vi "回正判定.vi"(0 "曲线引用":refnum<vi>, 1 "回正判定":T1, 3 "错误输入":errorcluster) -> (7 "曲线引用输出":refnum<vi>, 8 "OK":bool, 10 "错误输出":errorcluster)   [LabVIEW 2018]
uses:
  Global_Variable/Global.vi
  Global_Variable/A180648.vi
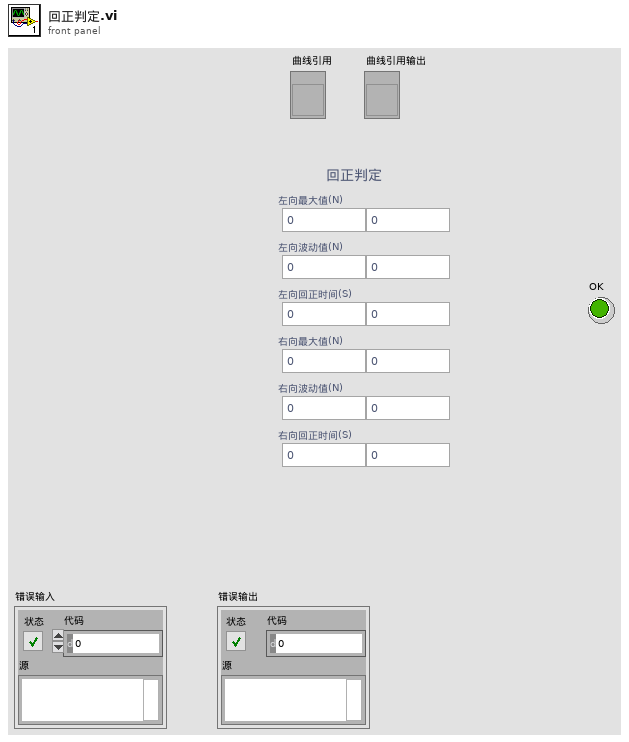
[diagram p1: front panel]
types:
  T1 = cluster{"左向最大值(N)":cluster{"下限":dbl, "上限":dbl}, "左向波动值(N)":cluster{"下限":dbl, "上限":dbl}, "左向回正时间(S)":cluster{"下限":dbl, "上限":dbl}, "右向最大值(N)":cluster{"下限":dbl, "上限":dbl}, "右向波动值(N)":cluster{"下限":dbl, "上限":dbl}, "右向回正时间(S)":cluster{"下限":dbl, "上限":dbl}}
  T2 = enum32{"空载", "功能", "力特性", "传感器特性", "电流特性", "振动NVH", "逆向空载", "完成"}
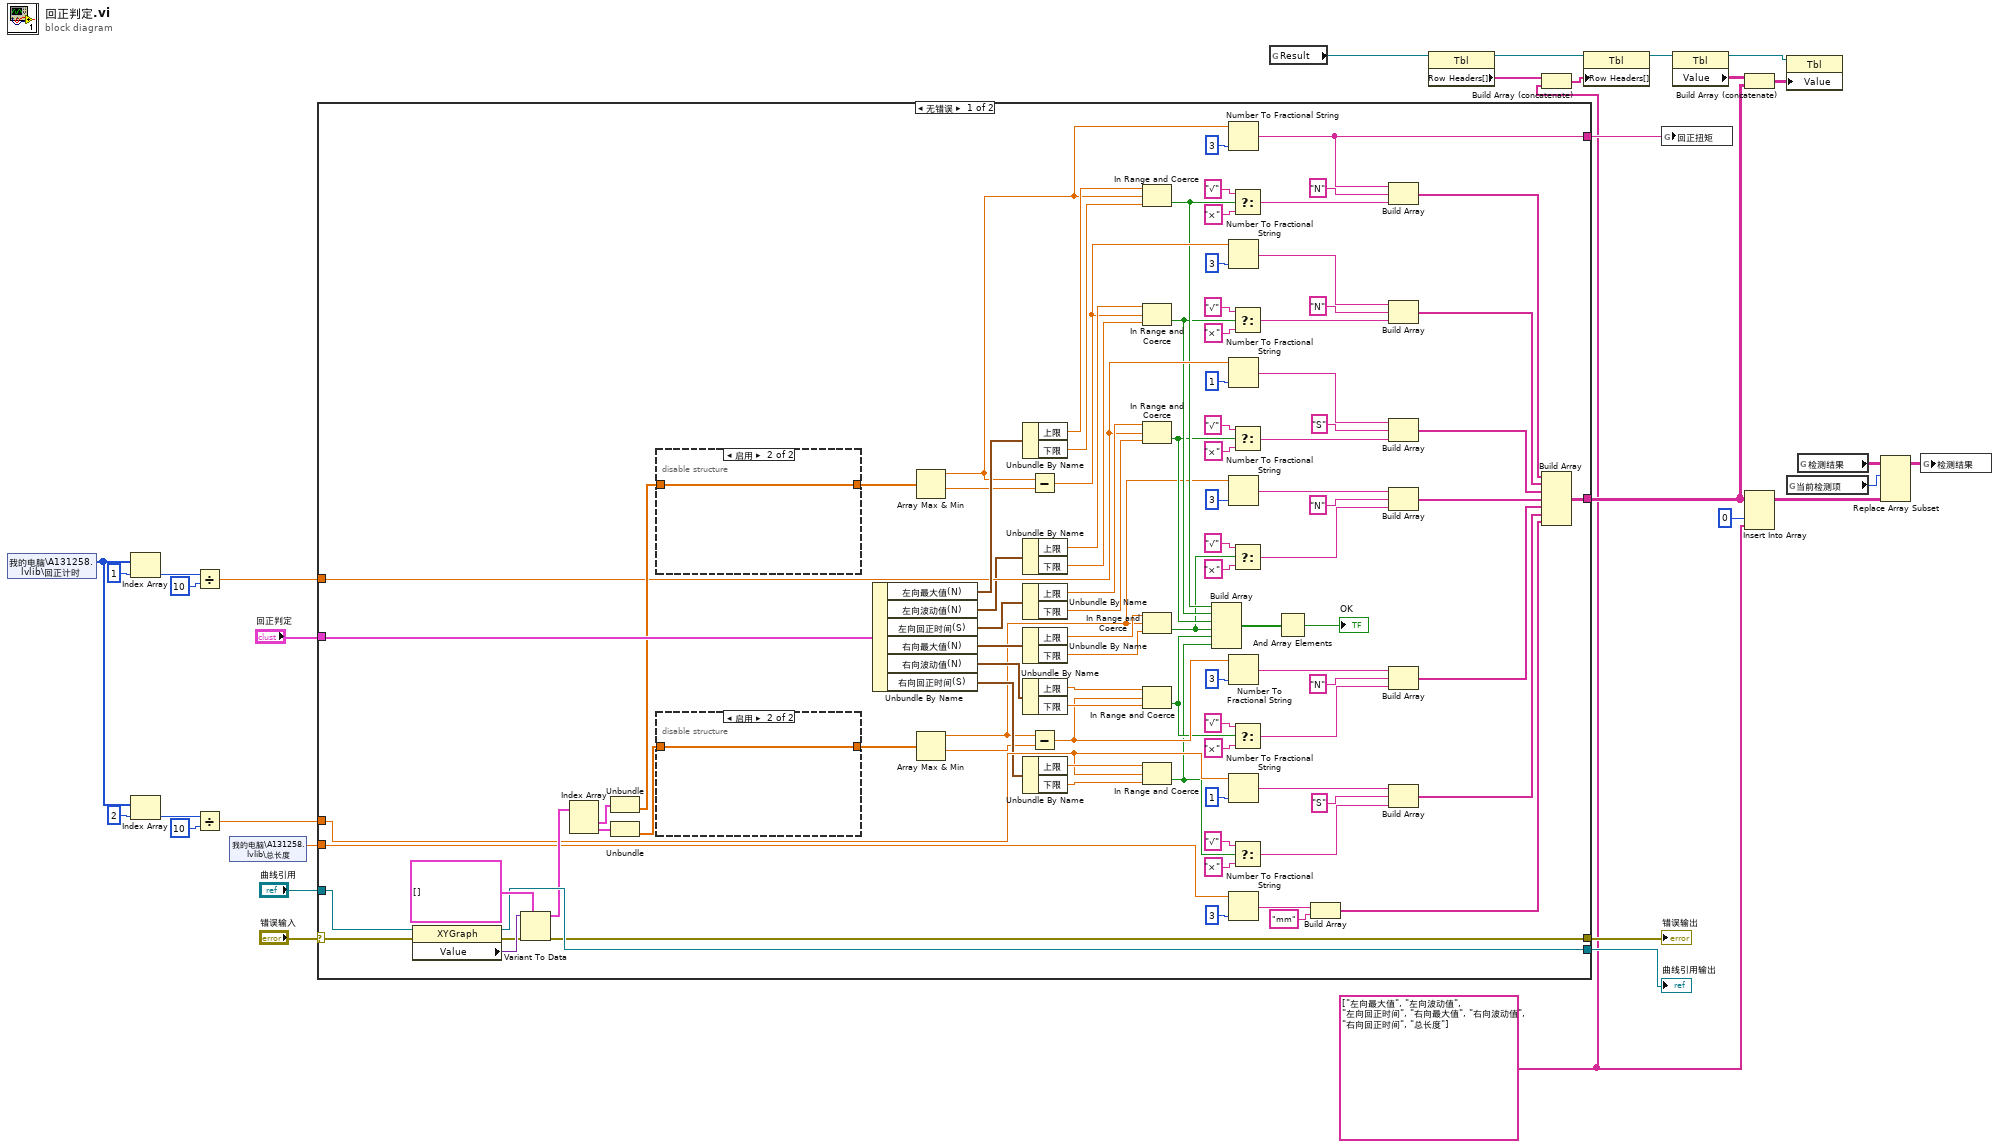
[diagram p0: block diagram]
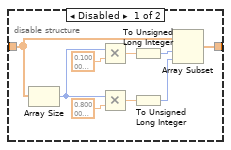
[diagram p2: hidden frame]
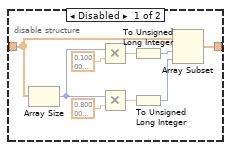
[diagram p3: hidden frame]
diagram:
  w3 = string[] ["左向最大值", "左向波动值", "左向回正时间", "右向最大值", "右向波动值", "右向回正时间", "总长度"] ("元素")
  n1 = shared-variable "我的电脑\\A131258.lvlib\\回正计时"() -> (w15:u32[])  [unwired: 1 in, 1 out]
  n2 = Index Array(array=w15, index=1 ("索引")) -> (element=w13:u32)
  n3 = Index Array(array=w15, index=2 ("索引")) -> (element=w10:u32)
  n4 = Divide(x=w13, y=u32 10) -> (x/y=w14:dbl)
  n5 = Divide(x=w10, y=u32 10) -> (x/y=w9:dbl)
  n6 = shared-variable "我的电脑\\A131258.lvlib\\总长度"() -> (w8:sgl)  [unwired: 1 in, 1 out]
  n7 = case shown="无错误" "错误输入" {
    selector: "错误输入" -> [w126 w150]
    tunnel: [w122 w150] -> w30
    tunnel: "曲线引用" -> [w125 w149]
    tunnel: [w124 w149] -> w28
    tunnel: "回正判定" -> [w118 _]
    tunnel: [w101 _] -> w4
    tunnel: [w96 _] -> w19
    tunnel: w14 -> [w55 _]
    tunnel: w9 -> [w54 _]
    tunnel: w8 -> [w34 _]
    frame No Error {
      n8 = property class="XYGraph"(reference=w125, error in=w126) -> (reference out=w124:refnum<vi>, error out=w123:errorcluster, "Value"=w128:variant)
      n9 = Variant To Data(error in=w123, type=cluster{dbl[], dbl[]}[] [], Variant=w128) -> (data=w121:cluster{dbl[], dbl[]}[], error out=w122:errorcluster)
      n10 = Index Array(array=w121) -> (element #1=w120:cluster{dbl[], dbl[]}, element #2=w119:cluster{dbl[], dbl[]})  [unwired: 2 in]
      n11 = Unbundle(w120) -> (w63:dbl[])  [unwired: 1 out]
      n12 = Unbundle(w119) -> (w62:dbl[])  [unwired: 1 out]
      n13 = disable-structure shown="启用" {
        disable-tunnel: [w147 w148] -> w99
        disable-tunnel: w63 -> [w139 w148]
        frame Disabled {
          n14 = Array Size(array=w139) -> (size(s)=w140:i32)
          n15 = Multiply(x=w140, y=sgl 0.1) -> (x*y=w144:sgl)
          n16 = Multiply(x=w140, y=sgl 0.8) -> (x*y=w145:sgl)
          n17 = To Unsigned Long Integer(number=w144) -> (unsigned 32bit integer=w146:u32)
          n18 = To Unsigned Long Integer(number=w145) -> (unsigned 32bit integer=w141:u32)
          n19 = Array Subset(array=w139, index=w146, length=w141) -> (w147:dbl[])
        }
        frame Enabled {
        }
      }
      n20 = disable-structure shown="启用" {
        disable-tunnel: [w137 w138] -> w100
        disable-tunnel: w62 -> [w129 w138]
        frame Disabled {
          n21 = Array Size(array=w129) -> (size(s)=w136:i32)
          n22 = Multiply(x=w136, y=sgl 0.1) -> (x*y=w132:sgl)
          n23 = Multiply(x=w136, y=sgl 0.8) -> (x*y=w131:sgl)
          n24 = To Unsigned Long Integer(number=w132) -> (unsigned 32bit integer=w130:u32)
          n25 = To Unsigned Long Integer(number=w131) -> (unsigned 32bit integer=w135:u32)
          n26 = Array Subset(array=w129, index=w130, length=w135) -> (w137:dbl[])
        }
        frame Enabled {
        }
      }
      n27 = Unbundle By Name(w118) -> ("左向最大值(N)"=w117:cluster{"下限":dbl, "上限":dbl}, "左向波动值(N)"=w53:cluster{"下限":dbl, "上限":dbl}, "左向回正时间(S)"=w52:cluster{"下限":dbl, "上限":dbl}, "右向最大值(N)"=w61:cluster{"下限":dbl, "上限":dbl}, "右向波动值(N)"=w51:cluster{"下限":dbl, "上限":dbl}, "右向回正时间(S)"=w50:cluster{"下限":dbl, "上限":dbl})
      n28 = Array Max & Min(array=w99) -> (max value=w60:dbl, min value=w59:dbl)  [unwired: 2 out]
      n29 = Array Max & Min(array=w100) -> (max value=w32:dbl, min value=w49:dbl)  [unwired: 2 out]
      n30 = Unbundle By Name(w117) -> ("上限"=w103:dbl, "下限"=w102:dbl)
      n31 = Unbundle By Name(w53) -> ("上限"=w93:dbl, "下限"=w94:dbl)
      n32 = Unbundle By Name(w52) -> ("上限"=w82:dbl, "下限"=w81:dbl)
      n33 = Unbundle By Name(w61) -> ("上限"=w98:dbl, "下限"=w97:dbl)
      n34 = Unbundle By Name(w51) -> ("上限"=w78:dbl, "下限"=w79:dbl)
      n35 = Unbundle By Name(w50) -> ("上限"=w65:dbl, "下限"=w64:dbl)
      n36 = Subtract(x=w60, y=w59) -> (x-y=w58:dbl)
      n37 = Subtract(x=w32, y=w49) -> (x-y=w48:dbl)
      n38 = In Range and Coerce(upper limit=w103, x=w60, lower limit=w102) -> (In Range?=w43:bool)  [unwired: 1 out]
      n39 = In Range and Coerce(upper limit=w93, x=w58, lower limit=w94) -> (In Range?=w42:bool)  [unwired: 1 out]
      n40 = In Range and Coerce(upper limit=w82, x=w55, lower limit=w81) -> (In Range?=w41:bool)  [unwired: 1 out]
      n41 = In Range and Coerce(upper limit=w98, x=w32, lower limit=w97) -> (In Range?=w40:bool)  [unwired: 1 out]
      n42 = In Range and Coerce(upper limit=w78, x=w48, lower limit=w79) -> (In Range?=w39:bool)  [unwired: 1 out]
      n43 = In Range and Coerce(upper limit=w65, x=w54, lower limit=w64) -> (In Range?=w38:bool)  [unwired: 1 out]
      n44 = Build Array(w43, w42, w41, w40, w39, w38) -> (w105:bool[])
      n45 = Number To Fractional String(number=w60, precision (6)=i16 3 ("精度(6)")) -> (F-format string=w96:string)  [unwired: 2 in]
      n46 = Number To Fractional String(number=w58, precision (6)=i16 3 ("精度(6)")) -> (F-format string=w95:string)  [unwired: 2 in]
      n47 = Number To Fractional String(number=w55, precision (6)=i16 1 ("精度(6)")) -> (F-format string=w80:string)  [unwired: 2 in]
      n48 = Number To Fractional String(number=w32, precision (6)=i16 3 ("精度(6)")) -> (F-format string=w107:string)  [unwired: 2 in]
      n49 = Number To Fractional String(number=w48, precision (6)=i16 3 ("精度(6)")) -> (F-format string=w76:string)  [unwired: 2 in]
      n50 = Number To Fractional String(number=w54, precision (6)=i16 1 ("精度(6)")) -> (F-format string=w67:string)  [unwired: 2 in]
      n51 = Number To Fractional String(number=w34, precision (6)=i16 3 ("精度(6)")) -> (F-format string=w36:string)  [unwired: 2 in]
      n52 = Select(t="√", s=w43, f="×") -> (s? t:f=w112:string)
      n53 = Select(t="√", s=w42, f="×") -> (s? t:f=w92:string)
      n54 = Select(t="√", s=w41, f="×") -> (s? t:f=w83:string)
      n55 = Select(t="√", s=w40, f="×") -> (s? t:f=w111:string)
      n56 = Select(t="√", s=w39, f="×") -> (s? t:f=w72:string)
      n57 = Select(t="√", s=w38, f="×") -> (s? t:f=w71:string)
      n58 = And Array Elements(Boolean array=w105) -> (logical AND=→"OK":bool)
      n59 = Build Array(w36, "mm" ("元素")) -> (w33:string[])
      n60 = Build Array(w96, "N" ("元素"), w112) -> (w57:string[])
      n61 = Build Array(w95, "N" ("元素"), w92) -> (w56:string[])
      n62 = Build Array(w80, "S" ("元素"), w83) -> (w47:string[])
      n63 = Build Array(w107, "N" ("元素"), w111) -> (w46:string[])
      n64 = Build Array(w76, "N" ("元素"), w72) -> (w45:string[])
      n65 = Build Array(w67, "S" ("元素"), w71) -> (w44:string[])
      n66 = Build Array(w57, w56, w47, w46, w45, w44, w33) -> (w101:string[][])
    }
    frame Error {
    }
  }
  "错误输出" <- w30
  "曲线引用输出" <- w28
  n67 = global read "Global.vi" "Result"() -> (w27:refnum<vi>)
  n68 = property class="Tbl"(reference=w27) -> (reference out=w24:refnum<vi>, "Row Headers[]"=w26:string[])  [unwired: 1 in, 1 out]
  n69 = Build Array (concatenate)(w26, w3) -> (w25:string[])
  n70 = property class="Tbl"(reference=w24, "Row Headers[]"=w25) -> (reference out=w23:refnum<vi>)  [unwired: 1 in, 1 out]
  n71 = global write "检测结果.vi" "回正扭矩"(w19) -> ()
  n72 = property class="Tbl"(reference=w23) -> (reference out=w22:refnum<vi>, "Value"=w21:string[][])  [unwired: 1 in, 1 out]
  n73 = Build Array (concatenate)(w21, w4) -> (w20:string[][])
  n74 = Insert Into Array(array=w4, index (col)=0 ("禁用的索引 (列)"), new element=w3) -> (w1:string[][])  [unwired: 1 in]
  n75 = property class="Tbl"(reference=w22, "Value"=w20) -> ()  [unwired: 1 in, 2 out]
  n76 = global read "A180648.vi" "当前检测项"() -> (w6:T2)
  n77 = global read "A180648.vi" "检测结果"() -> (w7:string[][][])
  n78 = Replace Array Subset(array=w7, new element=w1, index (dim 0)=w6) -> (w5:string[][][])  [unwired: 2 in]
  n79 = global write "A180648.vi" "检测结果"(w5) -> ()
